vi "set_stage_and_electrode_init (SubVI).vi"(8 "Flash lamp settings:":T1={"Output channel (for flashing)"="Dev4/ao0", "Loop iteration"=0, "Path"=path "", "Flash lamp\n settings:"={"Flash lamp?"=FALSE, "Number of cyles\nbetween flashes"=3, "# Pulses"=35, "Stop flashing \nbelow thresh?"=FALSE, "Stop threshold"=0.001, "Pulse voltage?"=FALSE, "Pulse length (ms)"=0.001, "Pulse amp (V)"=0.001}}, 9 "instrument config":T3, 10 "Process list":T2, 11 "Cluster in":refnum<vi>) -> (3 "Curr threshold":dbl)   [LabVIEW 2018]
uses:
  <vilib>/DAQmx/configure/trigger.llb/DAQmx Start Trigger (None).vi
  <resource>/objmgr/daqmx.rc
panel:
  out "init_display":dbl[][](graph)
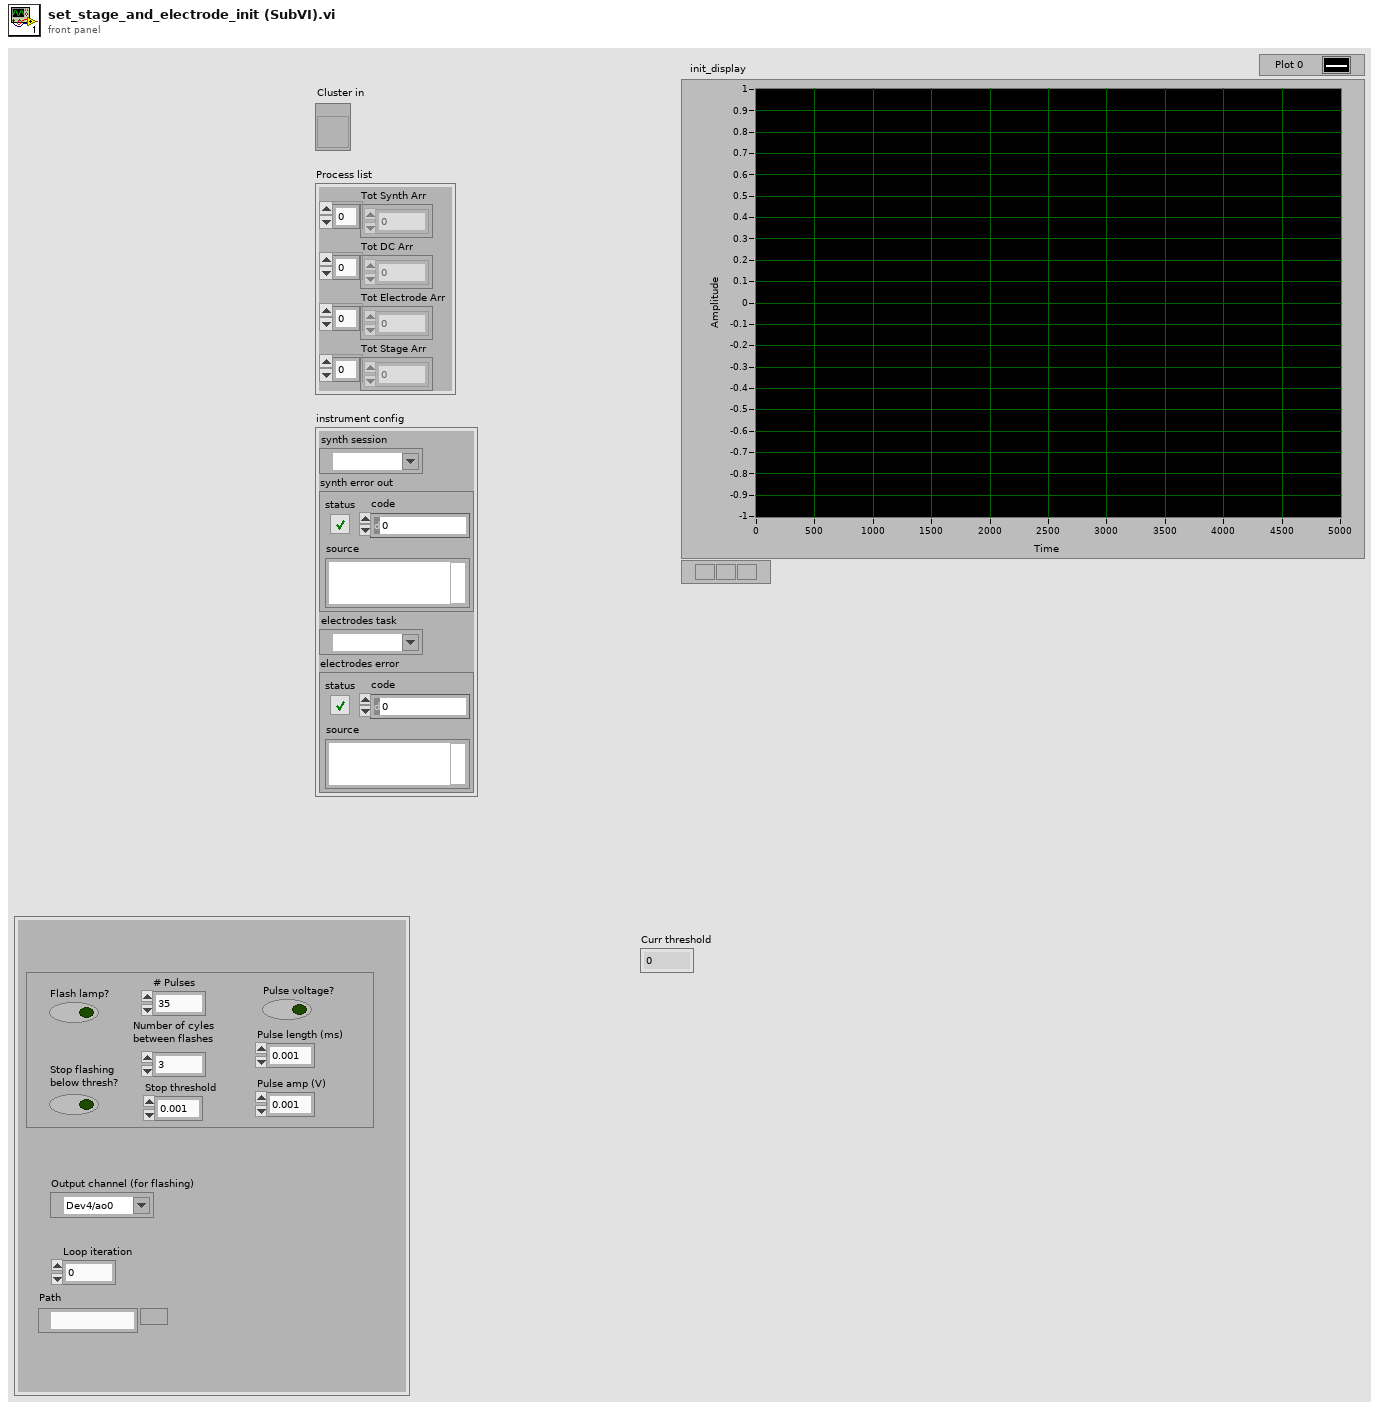
[diagram p1: front panel]
types:
  T1 = cluster{"Output channel (for flashing)":tag, "Loop iteration":i32, "Path":path, "Flash lamp\n settings:":cluster{"Flash lamp?":bool, "Number of cyles\nbetween flashes":i32, "# Pulses":i32, "Stop flashing \nbelow thresh?":bool, "Stop threshold":dbl, "Pulse voltage?":bool, "Pulse length (ms)":dbl, "Pulse amp (V)":dbl}}
  T2 = cluster{"Tot Synth Arr":dbl[], "Tot DC Arr":dbl[], "Tot Electrode Arr":dbl[], "Tot Stage Arr":dbl[]}
  T3 = cluster{"synth session":refnum<visa-resource-name>, "synth error out":errorcluster, "electrodes task":refnum<k21>, "electrodes error":errorcluster}
  T4 = cluster{"Flash lamp?":bool, "Number of cyles\nbetween flashes":i32, "# Pulses":i32, "Stop flashing \nbelow thresh?":bool, "Stop threshold":dbl, "Pulse voltage?":bool, "Pulse length (ms)":dbl, "Pulse amp (V)":dbl}
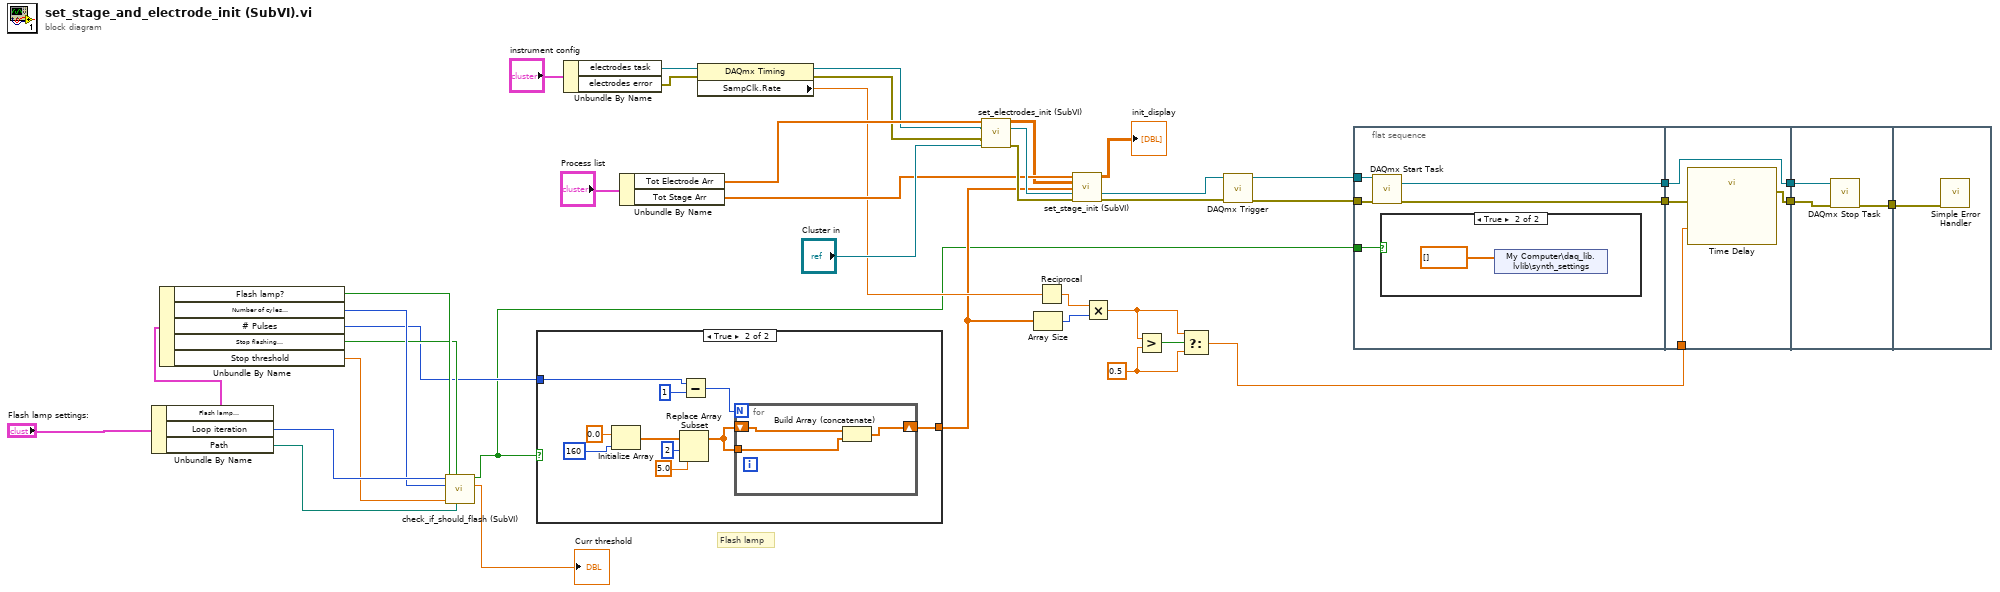
[diagram p0: block diagram]
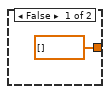
[diagram p2: hidden frame]
diagram:
  w3 = 0.5 ("element")
  # "Flash lamp"
  n1 = Unbundle By Name("Flash lamp settings:") -> ("Flash lamp\n settings:"=w21:T4, "Loop iteration"=w19:i32, "Path"=w20:path)
  n2 = Unbundle By Name(w21) -> ("Flash lamp?"=w16:bool, "Number of cyles\nbetween flashes"=w17:i32, "# Pulses"=w14:i32, "Stop flashing \nbelow thresh?"=w15:bool, "Stop threshold"=w18:dbl)
  n3 = call "check_if_should_flash (SubVI).vi"("Path"=w20, "Stop below threshold"=w15, "Stop threshold"=w18, "Flash lamp?"=w16, "Number of cyles\nbetween flashes"=w17, "Loop iteration"=w19) -> ("Curr threshold"=→"Curr threshold":dbl, "Should flash"=w1:bool)  [unwired: 4 in]
  n4 = case shown="True" w1 {
    tunnel: w14 -> [_ w44]
    tunnel: [dbl[] [] w43] -> w8
    frame False {
    }
    frame True {
      n5 = Initialize Array(0.0 ("element"), 160 ("y")) -> (w51:dbl[])
      n6 = Replace Array Subset(array=w51, new element=5.0 ("new element/subarray"), index=2) -> (w48:dbl[])
      n7 = Subtract(x=w44, y=1) -> (x-y=w52:i32)
      n8 = for {
        N: w52 -> [_]
        shift-right: [w53] -> w43
        shift-left: w48 -> [w55]
        tunnel: w48 -> [w54]
        n9 = Build Array (concatenate)(w55, w54) -> (w53:dbl[])
      }
    }
  }
  n10 = Unbundle By Name("instrument config") -> ("electrodes task"=w13:refnum<k21>, "electrodes error"=w12:errorcluster)
  n11 = Unbundle By Name("Process list") -> ("Tot Electrode Arr"=w36:dbl[], "Tot Stage Arr"=w38:dbl[])
  n12 = property class="DAQmx Timing"(reference=w13, error in=w12) -> (reference out=w11:refnum<k21>, error out=w10:errorcluster, "SampClk.Rate"=w9:dbl)
  n13 = call "set_electrodes_init (SubVI).vi"("Tot Electrode Arr"=w36, "electrodes task 2"=w11, "electrodes error"=w10, "electrodes reference"="Cluster in") -> ("electrode arr"=w37:dbl[][], "electrodes task"=w40:refnum<k21>, "electrodes task error"=w39:errorcluster)  [unwired: 9 in]
  n14 = Array Size(array=w8) -> (size(s)=w6:i32)
  n15 = Reciprocal(x=w9) -> (1/x=w7:dbl)
  n16 = call "set_stage_init (SubVI).vi"("Tot Stage Arr"=w38, "electrode arr"=w37, "flash_arr"=w8, "electrodes task"=w40, "electrodes task error"=w39) -> ("init_arr"=→"init_display":dbl[][], "electrodes task 2"=w31:refnum<k21>, "electrodes task error 2"=w30:errorcluster)  [unwired: 8 in]
  n17 = Multiply(x=w7, y=w6) -> (x*y=w4:dbl)
  n18 = Greater?(x=w4, y=w3) -> (0:w5:bool)
  n19 = Select(t=w4, s=w5, f=w3) -> (s? t:f=w2:dbl)
  n20 = call-poly <vilib>:"DAQmx Trigger.vi"("task/channels in"=w31, "error in"=w30) -> ("task out"=w33:refnum<k21>, "error out"=w32:errorcluster)  [unwired: 12 in]
  n21 = flat-sequence {
    tunnel: w33 -> [w60]
    tunnel: w32 -> [w59]
    tunnel: [w58] -> w28
    tunnel: [w57] -> w26
    tunnel: w1 -> [w56]
    tunnel: w28 -> [w63]
    tunnel: [w63] -> w27
    tunnel: w26 -> [w65]
    tunnel: [w64] -> w25
    tunnel: w2 -> [w62]
    tunnel: w27 -> [w68]
    tunnel: w25 -> [w67]
    tunnel: [w66] -> w29
    tunnel: w29 -> [w69]
    frame #0 {
      n22 = call <vilib>:"DAQmx Start Task.vi"("task/channels in"=w60, "error in"=w59) -> ("task out"=w58:refnum<k21>, "error out"=w57:errorcluster)  [unwired: 12 in]
      n23 = case shown="True" w56 {
        frame False {
        }
        frame True {
          n24 = shared-variable "My Computer\\daq_lib.lvlib\\synth_settings"(dbl[] [] ("appended array")) -> ()  [unwired: 1 in, 1 out]
        }
      }
    }
    frame #1 {
      n25 = call "Time Delay"("error in (no error)"=w65, "Delay Time (s)"=w62) -> ("error out"=w64:errorcluster)  [unwired: 9 in]
    }
    frame #2 {
      n26 = call <vilib>:"DAQmx Stop Task.vi"("task/channels in"=w68, "error in"=w67) -> ("error out"=w66:errorcluster)  [unwired: 12 in, 1 out]
    }
    frame #3 {
      n27 = call <vilib>:"Simple Error Handler.vi"("error in (no error)"=w69) -> ()  [unwired: 4 in, 5 out]
    }
  }
